vi "Template_StateMachine.vi"() -> ()   [LabVIEW 2026]
doc: "Illustre les principes de base du modèle de conception de machine à états dans LabVIEW. Les machines à états les plus simples sont composées d'une structure Condition dans une boucle While, avec un énum d'états câblé à un registre à décalage de la boucle pour définir l'exécution des différentes conditions (ou \"états\") de la structure Condition à différentes itérations de la boucle."
uses:
  Etats.ctl
panel:
  out "error out":errorcluster caption="sortie d'erreur"
  in  "error in":errorcluster caption="entrée d'erreur"
  in  "Arrêter":bool
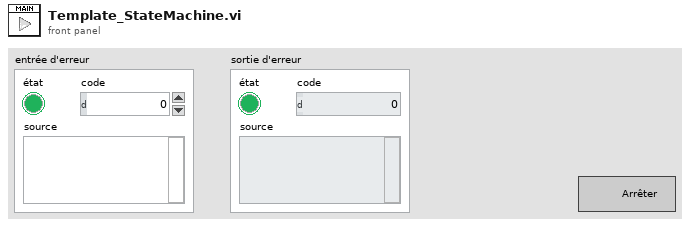
[diagram p1: front panel]
types:
  T1 = typedef "Etats.ctl" = enum16{"Init", "Stop", "Wait for Event", "Config"}
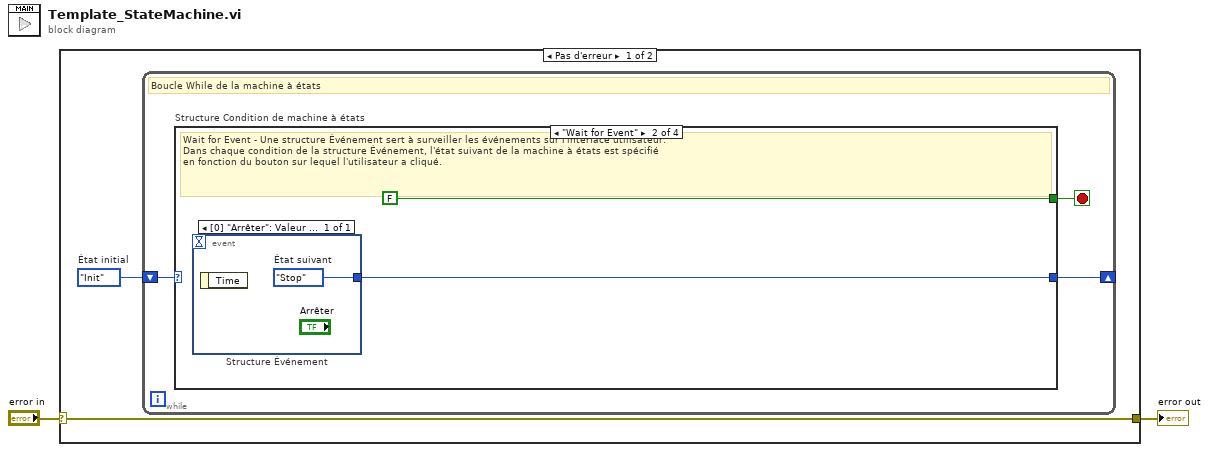
[diagram p0: block diagram]
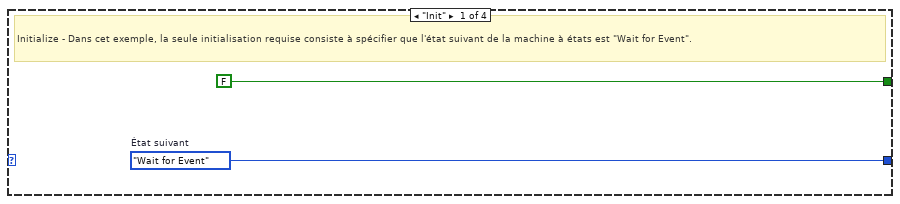
[diagram p2: hidden frame]
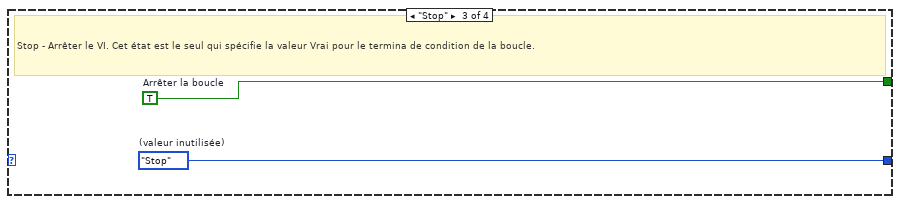
[diagram p3: hidden frame]
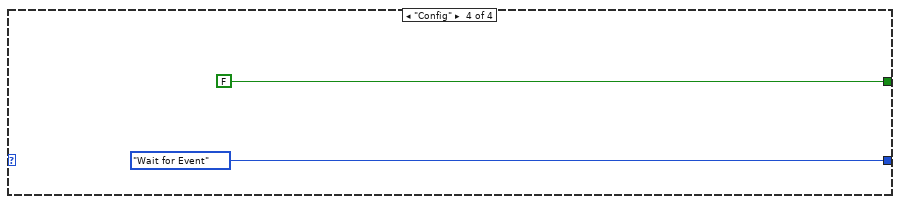
[diagram p4: hidden frame]
diagram:
  n1 = case shown="Pas d'erreur" "error in" {
    selector: "error in" -> [w3 w17]
    tunnel: [w3 w17] -> w1
    frame No Error {
      w4 = Etats."Init"  # État initial
      n2 = while {
        shift-right: [w6] -> _
        shift-left: w4 -> [w7]
        stop <- w5 stop-if-true
        # "Boucle While de la machine à états"
        n3 = case "Structure Condition de machine à états" shown="\"Wait for Event\"" w7 {
          tunnel: [w9 w11 w14 Etats."Wait for Event" ("(valeur inutilisée)")] -> w6
          tunnel: [FALSE ("Arrêter la boucle") FALSE ("Arrêter la boucle") w13 FALSE ("Arrêter la boucle")] -> w5
          frame "Init" {
            w9 = Etats."Wait for Event"  # État suivant
            # "Initialize - Dans cet exemple, la seule initialisation requise consiste à spécifier que l'état suivant de la machine à états est \"Wait for Event\"."
          }
          frame "Wait for Event" {
            # "Wait for Event - Une structure Événement sert à surveiller les événements sur l'interface utilisateur.\nDans chaque condition de la structure Événement, l'état suivant de la machine à états est spécifié\nen fonction du bouton sur lequel l'utilisateur a cliqué."
            n4 = event "Structure Événement" shown="[0] \"Arrêter\": Valeur changée" {
              selector: _ -> [_]
              dyn-events: _ -> [_]
              timeout: _ -> [_]
              tunnel: [w12] -> w11
              event "Arrêter": Value Change {
                w12 = Etats."Stop"  # État suivant
                n5 = event-data() -> ()  [unwired: 1 in, 1 out]
              }
            }
          }
          frame "Stop" {
            w13 = TRUE  # Arrêter la boucle
            w14 = Etats."Stop"  # (valeur inutilisée)
            # "Stop - Arrêter le VI. Cet état est le seul qui spécifie la valeur Vrai pour le termina de condition de la boucle."
          }
          frame "Config" {
          }
        }
      }
    }
    frame Error {
    }
  }
  "error out" <- w1
